vi "getNewValueXML.vi"(8 "error in (no error)":errorcluster, 11 "SingleToneRamp in":refnum<class "SingleToneRamp.lvclass">) -> (0 "error out":errorcluster, 2 "newValueXML":refnum<class "xmlNode.lvclass">, 3 "SingleToneRamp out":refnum<class "SingleToneRamp.lvclass">)   [LabVIEW 2011, in "Tools.lvlib" / "Scripting.lvlib" / "SingleToneRamp.lvclass"]
uses:
  SingleToneRamp.lvclass
  xmlNode/xmlNode.lvclass
  ScriptEvent.lvclass
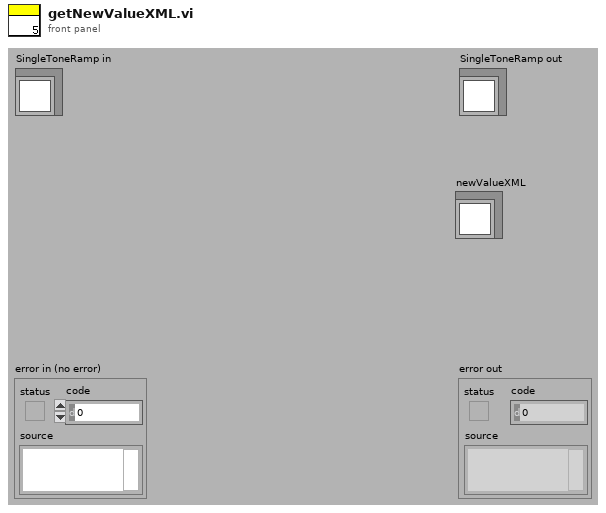
[diagram p1: front panel]
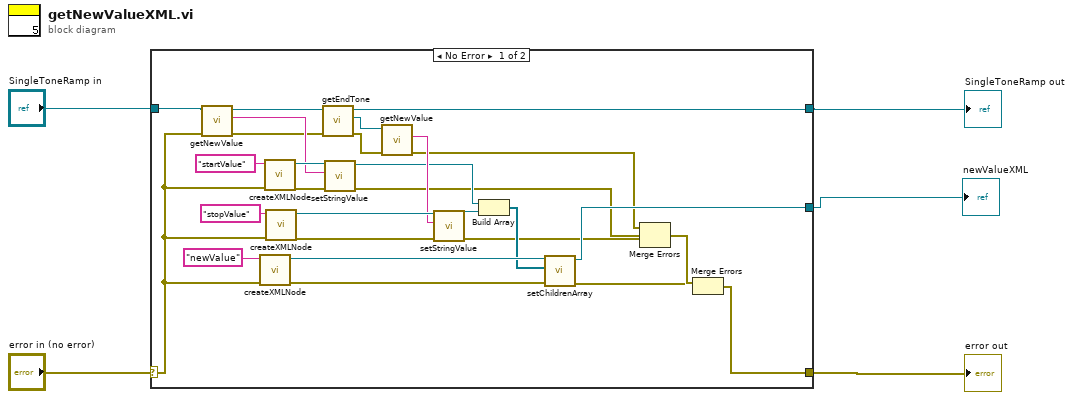
[diagram p0: block diagram]
diagram:
  n1 = case shown="No Error" "error in (no error)" {
    selector: "error in (no error)" -> [w29 w35]
    tunnel: [w11 w35] -> w2
    tunnel: [w9 w34] -> w4
    tunnel: "SingleToneRamp in" -> [w32 w34]
    tunnel: [w20 _] -> w1
    frame No Error {
      n2 = call "getNewValue.vi"("error in (no error)"=w29, "ScriptEvent.lvclass in"=w32) -> ("error out"=w6:errorcluster, "newValue"=w26:string, "ScriptEvent.lvclass out"=w10:refnum<class "SingleToneRamp.lvclass">)  [unwired: 7 in]
      n3 = call "createXMLNode.vi"("error in (no error)"=w29, "name"="newValue") -> ("error out"=w21:errorcluster, "xmlNode out"=w22:refnum<class "xmlNode.lvclass">)  [unwired: 8 in]
      n4 = call "createXMLNode.vi"("error in (no error)"=w29, "name"="startValue") -> ("error out"=w27:errorcluster, "xmlNode out"=w28:refnum<class "xmlNode.lvclass">)  [unwired: 8 in]
      n5 = call "createXMLNode.vi"("error in (no error)"=w29, "name"="stopValue") -> ("error out"=w24:errorcluster, "xmlNode out"=w25:refnum<class "xmlNode.lvclass">)  [unwired: 8 in]
      n6 = call "getEndTone.vi"("error in (no error)"=w6, "SingleToneRamp.lvclass in"=w10) -> ("error out"=w7:errorcluster, "endTone"=w8:refnum<class "SingleTone.lvclass">, "SingleToneRamp.lvclass out"=w9:refnum<class "SingleToneRamp.lvclass">)  [unwired: 7 in]
      n7 = call-dynamic "setStringValue.vi"("error in (no error)"=w27, "stringValue"=w26, "xmlNode.lvclass in"=w28) -> ("error out"=w15:errorcluster, "xmlNode.lvclass out"=w19:refnum<class "xmlNode.lvclass">)  [unwired: 7 in]
      n8 = call "getNewValue.vi"("error in (no error)"=w7, "ScriptEvent.lvclass in"=w8) -> ("error out"=w16:errorcluster, "newValue"=w23:string)  [unwired: 7 in, 1 out]
      n9 = call-dynamic "setStringValue.vi"("error in (no error)"=w24, "stringValue"=w23, "xmlNode.lvclass in"=w25) -> ("error out"=w14:errorcluster, "xmlNode.lvclass out"=w18:refnum<class "xmlNode.lvclass">)  [unwired: 7 in]
      n10 = Build Array(w19, w18) -> (w17:refnum<class "xmlNode.lvclass">[])
      n11 = call-dynamic "setChildrenArray.vi"("error in (no error)"=w21, "Children"=w17, "xmlNode.lvclass in"=w22) -> ("error out"=w12:errorcluster, "xmlNode.lvclass out"=w20:refnum<class "xmlNode.lvclass">)  [unwired: 7 in]
      n12 = Merge Errors(w16, w15, w14) -> (w13:errorcluster)
      n13 = Merge Errors(w13, w12) -> (w11:errorcluster)
    }
    frame Error {
    }
  }
  "error out" <- w2
  "SingleToneRamp out" <- w4
  "newValueXML" <- w1
